vi "pico_stringtoctls.vi"(10 "String in":string) -> (0 "aDir":bool=TRUE, 1 "response?":bool=TRUE, 2 "APulses":u16=300, 3 "APulsesButton":bool, 4 "aStop":bool, 7 "MIRROR":u16=1, 8 "aRate":dbl=1370.408163265306 format="%.2f", 9 "ARateButton":bool)   [LabVIEW 2011]
uses:
  <vilib>/regexp/Match Regular Expression.xnode
panel:
  # "Picomotor String to Controls"
  # "This VI parses a string into pico control values for input into picomove programs"
  # "The strings accepted are:\nstop\nrate:XXXX  sets the rate to XXXX\ngo:XXXX:dir:chan:axis  where dir=cw or ccw, chan and axis are integers \n                                      moves chan,axis by XXXX in direction dir"
  # "Target Rate"
  # "Pulse RATE"
  # "Do # PULSES"
  # "DIRECTION"
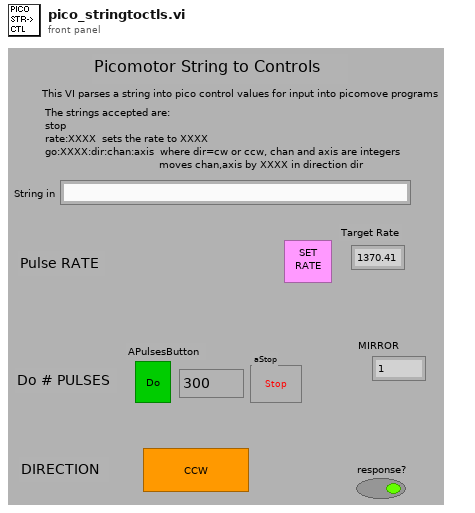
[diagram p1: front panel]
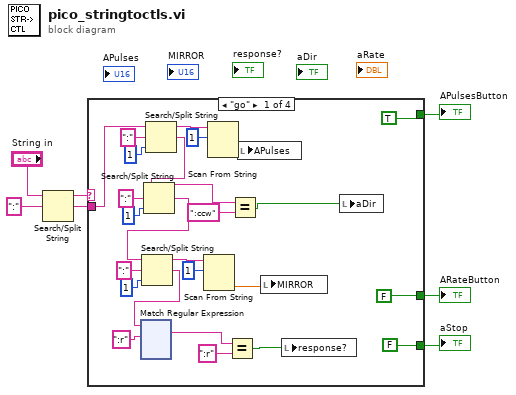
[diagram p0: block diagram]
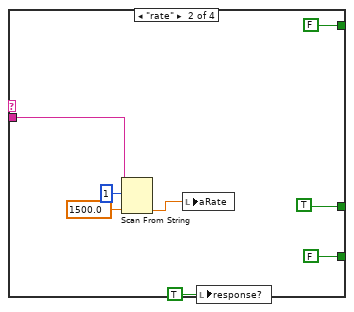
[diagram p2: hidden frame]
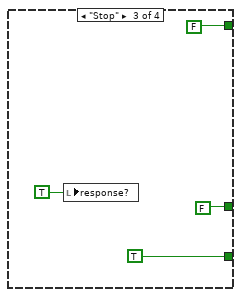
[diagram p3: hidden frame]
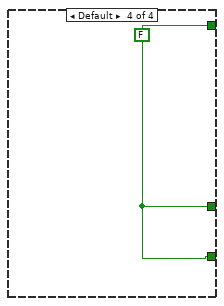
[diagram p4: hidden frame]
diagram:
  n1 = Search/Split String(string="String in", search string/char (-)=":") -> (substring before match=w5:string, match + rest of string=w4:string)  [unwired: 2 out]
  n2 = case shown="\"go\"" w5 {
    tunnel: w4 -> [w28 w150 _ _]
    tunnel: [FALSE ("aStop") FALSE ("aStop") TRUE ("aStop") w158] -> w3
    tunnel: [FALSE ("aStop") TRUE ("aStop") FALSE ("aStop") w158] -> w2
    tunnel: [TRUE ("aStop") FALSE ("aStop") FALSE ("aStop") w158] -> w1
    frame "go" {
      n3 = Search/Split String(string=w28, search string/char (-)=":", offset (0)=1) -> (substring before match=w26:string, match + rest of string=w18:string)  [unwired: 1 out]
      n4 = Search/Split String(string=w18, search string/char (-)=":", offset (0)=1) -> (substring before match=w15:string, match + rest of string=w17:string)  [unwired: 1 out]
      n5 = Search/Split String(string=w17, search string/char (-)=":", offset (0)=1) -> (substring before match=w19:string, match + rest of string=w8:string)  [unwired: 1 out]
      n6 = xnode "Match Regular Expression"("input string"=w8, "regular expression"=":r" ("search string/char (-)")) -> ("whole match"=w9:string)  [unwired: 3 in, 5 out]
      n7 = Scan From String(input string=w19, initial scan location=u32 1) -> (output 1=w16:dbl)  [unwired: 2 in, 4 out]
      n8 = Scan From String(input string=w26, initial scan location=u32 1) -> (output 1=w25:dbl)  [unwired: 2 in, 4 out]
      n9 = Equal?(x=w9, y=":r") -> (x = y?=w10:bool)
      n10 = Equal?(x=w15, y=":ccw") -> (x = y?=w13:bool)
      n11 = local write "APulses"(w25) -> ()
      n12 = local write "MIRROR"(w16) -> ()
      n13 = local write "response?"(w10) -> ()
      n14 = local write "aDir"(w13) -> ()
    }
    frame "rate" {
      n15 = Scan From String(input string=w150, initial scan location=u32 1, default 1=1500.0 ("default value 1")) -> (output 1=w147:dbl)  [unwired: 2 in, 3 out]
      n16 = local write "aRate"(w147) -> ()
      n17 = local write "response?"(TRUE ("response?")) -> ()
    }
    frame "Stop" {
      n18 = local write "response?"(TRUE ("response?")) -> ()
    }
    frame Default {
      w158 = FALSE ("aStop")
      n19 = local write "response?"(FALSE ("response?")) -> ()
    }
  }
  "APulsesButton" <- w1
  "ARateButton" <- w2
  "aStop" <- w3
